vi "Wave1D_Init Data.vi"(5 "Initial Derivative":dbl[](array[numeric]), 6 "Boundary Condition":cluster{"type":T2, "Value":dbl[]}[](array[cluster]) {"type" items=["Dirichlet", "Neumann"]}, 7 "Initial Value":dbl[](array[numeric]), 8 "Domain":T4={"t"={"initial t"=0.0, "final t"=1.0, "# of t-points"=11}, "x"={"start x"=0.0, "end x"=1.0, "# of x-points"=11}}, 9 "a":dbl, 10 "k":dbl=1.0, 11 "F(t, x)":dbl[][](array[numeric])) -> (3 "Wave1D Data":T1 {"BC"."End X"."type" items=["Dirichlet", "Neumann"]; "BC"."Start X"."type" items=["Dirichlet", "Neumann"]})   [LabVIEW 2020, in "NI_PDE.lvlib"]
uses:
  <vilib>/gmath/NI_PDE.lvlib
  <vilib>/gmath/pde.llb/Common/PDE_BC Type.ctl
  <vilib>/gmath/pde.llb/Wave1D/Wave1D_Data.ctl
  <vilib>/Analysis/Matrix/Datatypes/RealMatrix.ctl
  <vilib>/Analysis/Matrix/NI_Matrix.lvlib
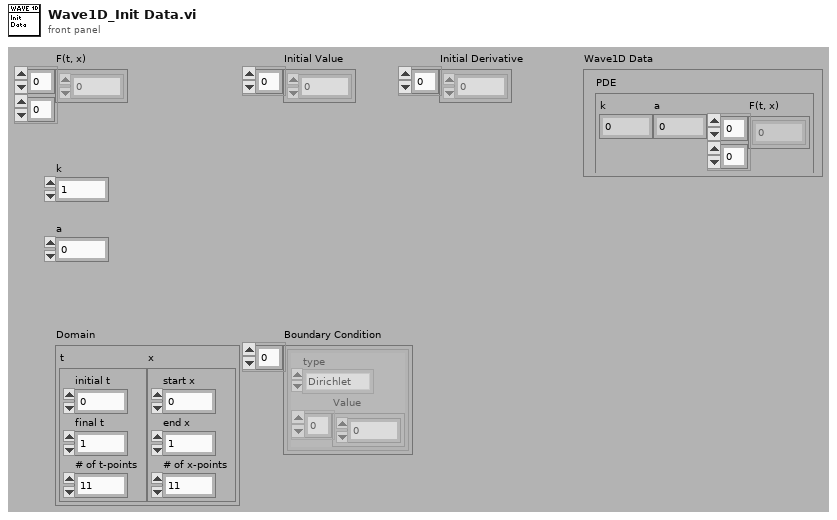
[diagram p1: front panel]
types:
  T1 = typedef "NI_PDE.lvlib/Wave1D_Data.ctl" = cluster{"PDE":cluster{"k":dbl, "a":dbl, "F(t, x)":dbl[][]}, "Domain":cluster{"t":cluster{"initial t":dbl, "final t":dbl, "# of t-points":i32}, "x":cluster{"start x":dbl, "end x":dbl, "# of x-points":i32}, "delta":cluster{"delta t":dbl, "delta x":dbl}}, "BC":cluster{"Start X":cluster{"type":T2, "Value":dbl[]}, "End X":cluster{"type":T2, "Value":dbl[]}}, "IC":cluster{"Value":dbl[], "Derivative":dbl[]}, "A":cluster{"Sub Diag":dbl[], "Diag":dbl[], "Super Diag":dbl[], "A":T3}, "LU of A":cluster{"L":dbl[], "U":cluster{"Diag":dbl[], "Super Diag":dbl[], "2nd Super Diag":dbl[]}, "Pivot":i32[]}, "State":cluster{"U":dbl[], "AU":dbl[], "Old AU":dbl[], "start index":i32, "length":i32}}
  T2 = typedef "NI_PDE.lvlib/PDE_BC Type.ctl" = i32
  T3 = typedef "NI_Matrix.lvlib/RealMatrix.ctl" = dbl[][]
  T4 = cluster{"t":cluster{"initial t":dbl, "final t":dbl, "# of t-points":i32}, "x":cluster{"start x":dbl, "end x":dbl, "# of x-points":i32}}
  T5 = cluster{"Start X":cluster{"type":T2, "Value":dbl[]}, "End X":cluster{"type":T2, "Value":dbl[]}}
  T6 = cluster{"L":dbl[], "U":cluster{"Diag":dbl[], "Super Diag":dbl[], "2nd Super Diag":dbl[]}, "Pivot":i32[]}
  T7 = cluster{"Sub Diag":dbl[], "Diag":dbl[], "Super Diag":dbl[], "A":T3}
  T8 = cluster{"initial t":dbl, "final t":dbl, "# of t-points":i32}
  T9 = cluster{"start x":dbl, "end x":dbl, "# of x-points":i32}
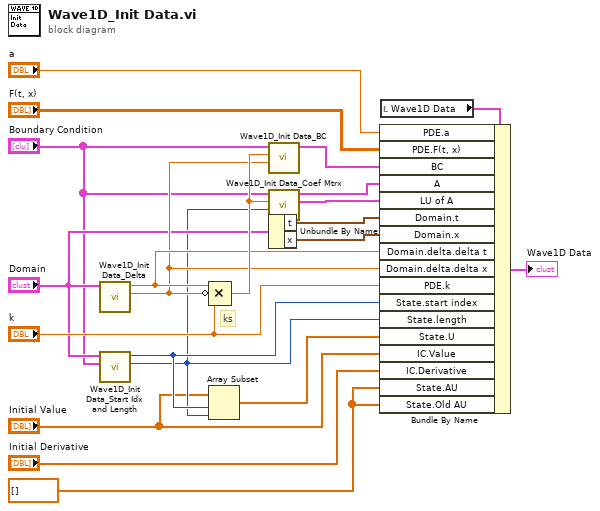
[diagram p0: block diagram]
diagram:
  w1 = dbl[] [] ("State.Old AU")
  # "ks"
  n1 = call <vilib>:"Wave1D_Init Data_Delta.vi"("Domain"="Domain") -> ("delta x"=w11:dbl, "delta t"=w12:dbl)  [unwired: 9 out]
  n2 = call <vilib>:"Wave1D_Init Data_Start Idx and Length.vi"("Boundary Condition"="Boundary Condition", "Domain"="Domain") -> ("length"=w6:i32, "start index"=w7:i32)  [unwired: 8 out]
  n3 = Compound Arithmetic op=MULTIPLY(w12, invert w11, "k") -> (w19:dbl)
  n4 = Array Subset(array="Initial Value", index=w7, length=w6) -> (w3:dbl[])
  n5 = call <vilib>:"Wave1D_Init Data_BC.vi"("delta x"=w11, "ks"=w19, "Boundary Condition"="Boundary Condition") -> ("BC"=w17:T5)  [unwired: 8 out]
  n6 = call <vilib>:"Wave1D_Init Data_Coef Mtrx.vi"("length"=w6, "ks"=w19, "Boundary Condition"="Boundary Condition") -> ("LU of A"=w20:T6, "A"=w18:T7)  [unwired: 7 out]
  n7 = Unbundle By Name("Domain") -> ("t"=w16:T8, "x"=w15:T9)
  n8 = local read "Wave1D Data"() -> (w21:T1)
  n9 = Bundle By Name(cluster=w21, "PDE.a"="a", "PDE.F(t, x)"="F(t, x)", "BC"=w17, "A"=w18, "LU of A"=w20, "Domain.t"=w16, "Domain.x"=w15, "Domain.delta.delta t"=w12, "Domain.delta.delta x"=w11, "PDE.k"="k", "State.start index"=w7, "State.length"=w6, "State.U"=w3, "IC.Value"="Initial Value", "IC.Derivative"="Initial Derivative", "State.AU"=w1, "State.Old AU"=w1) -> (→"Wave1D Data":T1)
